vi "44xx_AO_MinMax.vi"(9 "AO.channels":tag, 10 "AO.Range":T2) -> (1 "DAQ Type":T1, 2 "AO.max":dbl, 3 "AO.min":dbl)   [LabVIEW 2016, in "Instrument.Lockin.lvclass"]
uses:
  Instrument.Lockin.lvclass
  Typedefs/446xAO-enum.ctl
  Typedefs/DAQType-enum.ctl
  <resource>/objmgr/daqmx.rc
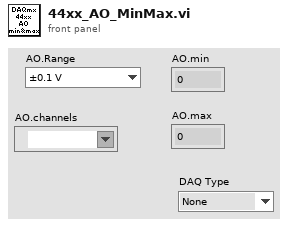
[diagram p1: front panel]
types:
  T1 = typedef "Instrument.Lockin.lvclass/DAQType-enum.ctl" = enum16{"None", "USB 4431", "PXI 446x"}
  T2 = typedef "Instrument.Lockin.lvclass/446xAO-enum.ctl" = enum16{"±0.1 V", "±1.0 V", "±10.0 V"}
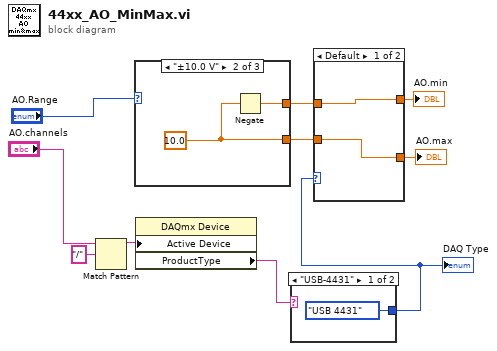
[diagram p0: block diagram]
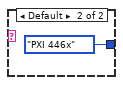
[diagram p2: hidden frame]
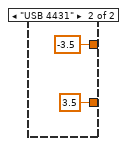
[diagram p3: hidden frame]
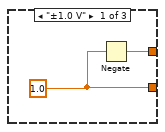
[diagram p4: hidden frame]
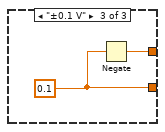
[diagram p5: hidden frame]
diagram:
  n1 = Match Pattern(string="AO.channels", regular expression="/") -> (before substring=w9:string)  [unwired: 1 in, 3 out]
  n2 = case shown="\"±10.0 V\"" "AO.Range" {
    tunnel: [w12 w14 w16] -> w3
    tunnel: [w11 w13 w15] -> w5
    frame "±1.0 V" {
      w12 = 1.0
      n3 = Negate(x=w12) -> (-x=w11:dbl)
    }
    frame "±10.0 V" {
      w14 = 10.0
      n4 = Negate(x=w14) -> (-x=w13:dbl)
    }
    frame "±0.1 V" {
      w16 = 0.1
      n5 = Negate(x=w16) -> (-x=w15:dbl)
    }
  }
  n6 = property class="DAQmx Device"("Active Device"=w9) -> ("ProductType"=w2:string)  [unwired: 2 in, 2 out]
  n7 = case shown="\"USB-4431\"" w2 {
    tunnel: [DAQType-enum."USB 4431" ("DAQ Type") DAQType-enum."PXI 446x" ("DAQ Type")] -> w1
    frame "USB-4431" {
    }
    frame Default {
    }
  }
  "DAQ Type" <- w1
  n8 = case shown="Default" w1 {
    tunnel: [w20 -3.5] -> w6
    tunnel: w5 -> [w20 _]
    tunnel: [w19 3.5] -> w4
    tunnel: w3 -> [w19 _]
    frame Default {
    }
    frame "USB 4431" {
    }
  }
  "AO.min" <- w6
  "AO.max" <- w4
